vi "Overwrite-all-variables.vi"(8 "error in (no error)":errorcluster, 10 "Analys. vars.":T1, 11 "Analysis params. ref. in":refnum<data-value>) -> (0 "error out":errorcluster, 3 "Analysis params. ref.":refnum<data-value>)   [LabVIEW 2013, in "CameraVision.lvlib" / "CV-Analysis.lvclass"]
uses:
  CV-Analysis.lvclass
  Analysis-variables.ctl
  Characteristics-cluster.ctl
  CV-Analysis.lvclass/CV-Analysis.ctl
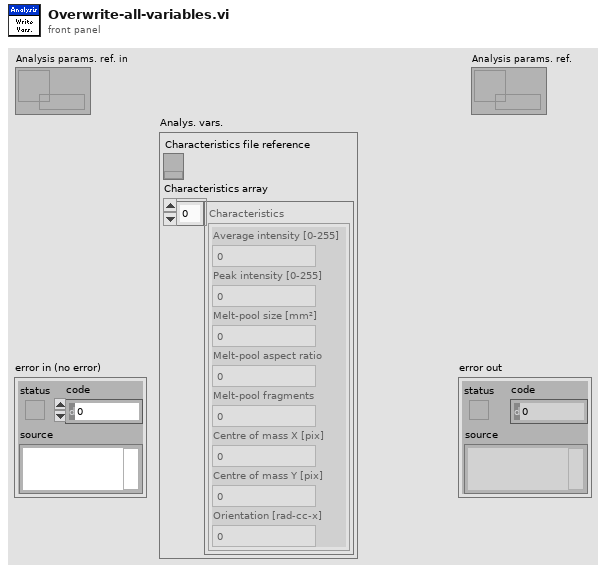
[diagram p1: front panel]
types:
  T1 = typedef "CameraVision.lvlib/CV-Analysis.lvclass/Analysis-variables.ctl" = cluster{"Characteristics file reference":refnum<k34>, "Characteristics array":T2[]}
  T2 = typedef "CameraVision.lvlib/CV-Analysis.lvclass/Characteristics-cluster.ctl" = cluster{"Average intensity":dbl, "Peak intensity":dbl, "Melt-pool size":dbl, "Melt-pool aspect ratio":dbl, "Melt-pool fragments":dbl, "Centre of mass X":dbl, "Centre of mass Y":dbl, "Orientation":dbl}
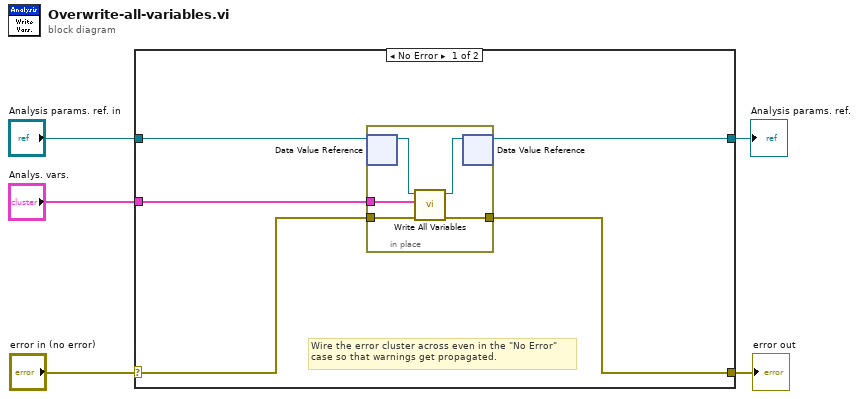
[diagram p0: block diagram]
diagram:
  n1 = case shown="No Error" "error in (no error)" {
    selector: "error in (no error)" -> [w9 w17]
    tunnel: [w10 w17] -> w4
    tunnel: "Analysis params. ref. in" -> [w8 w16]
    tunnel: "Analys. vars." -> [w6 _]
    tunnel: [w7 w16] -> w1
    frame No Error {
      # "Wire the error cluster across even in the \"No Error\"\ncase so that warnings get propagated."
      n2 = in-place {
        in-place-border: [w15] -> w10
        in-place-border: w9 -> [w14]
        in-place-border: w6 -> [w13]
        n3 = in-place-dvr #1(w8) -> (w12:refnum<class "CV-Analysis.lvclass">)  [unwired: 1 out]
        n4 = call "Write All Variables.vi"("error in (no error)"=w14, "Analys. vars."=w13, "Analysis params in"=w12) -> ("error out"=w15:errorcluster, "Analysis params out"=w11:refnum<class "CV-Analysis.lvclass">)  [unwired: 7 in]
        n5 = in-place-dvr #1(w11) -> (w7:refnum<data-value>)  [unwired: 1 out]
      }
    }
    frame Error {
    }
  }
  "error out" <- w4
  "Analysis params. ref." <- w1
